vi "Replace Line.vi"(8 "error in":errorcluster, 9 "New Line":T1 {"OPC UA Data Type" items=["Boolean"=1, "SByte"=2, "Byte"=3, "Int16"=4, "UInt16"=5, "Int32"=6, "UInt32"=7, "Int64"=8, "UInt64"=9, "Float"=10, "Double"=11, "String"=12, "DateTime"=13, "ByteString"=15, "Array of Boolean"=101, "Array of SByte"=102, "Array of Byte"=103, "Array of Int16"=104, "Array of UInt16"=105, "Array of Int32"=106, "Array of UInt32"=107, "Array of Int64"=108, "Array of UInt64"=109, "Array of Float"=110, "Array of Double"=111, "Array of String"=112, "Array of DateTime"=113, "Array of ByteString"=115]}, 10 "Line Name":string, 11 "OPC UA configuration in":refnum<class "OPC UA Client configuration.lvclass">) -> (0 "error out":errorcluster, 2 "Old Line":T1 {"OPC UA Data Type" items=["Boolean"=1, "SByte"=2, "Byte"=3, "Int16"=4, "UInt16"=5, "Int32"=6, "UInt32"=7, "Int64"=8, "UInt64"=9, "Float"=10, "Double"=11, "String"=12, "DateTime"=13, "ByteString"=15, "Array of Boolean"=101, "Array of SByte"=102, "Array of Byte"=103, "Array of Int16"=104, "Array of UInt16"=105, "Array of Int32"=106, "Array of UInt32"=107, "Array of Int64"=108, "Array of UInt64"=109, "Array of Float"=110, "Array of Double"=111, "Array of String"=112, "Array of DateTime"=113, "Array of ByteString"=115]}, 3 "OPC UA configuration out":refnum<class "OPC UA Client configuration.lvclass">)   [LabVIEW 2014, in "OPC UA Client configuration.lvclass"]
uses:
  OPC UA Client configuration.lvclass
  Line.ctl
  <vilib>/NI/Tag Bus Module Framework/channel/TBM channel.lvclass
  OPC UA Data Type.ctl
  OPC UA Client configuration.lvclass/OPC UA Client configuration.ctl
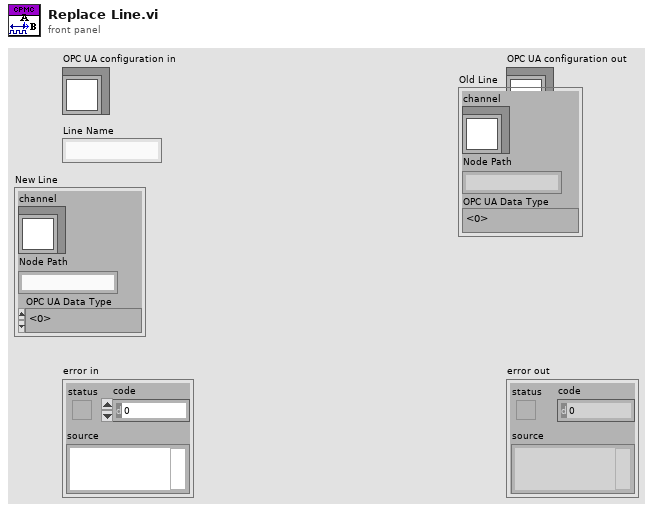
[diagram p1: front panel]
types:
  T1 = typedef "OPC UA Client configuration.lvclass/Line.ctl" = cluster{"channel":refnum<class "TBM channel.lvclass">, "Node Path":string, "OPC UA Data Type":T2}
  T2 = typedef "OPC UA Client configuration.lvclass/OPC UA Data Type.ctl" = u16
  T3 = cluster{"channel":refnum<class "TBM channel.lvclass">, "Node Path":string, "OPC UA Data Type":T2}[]
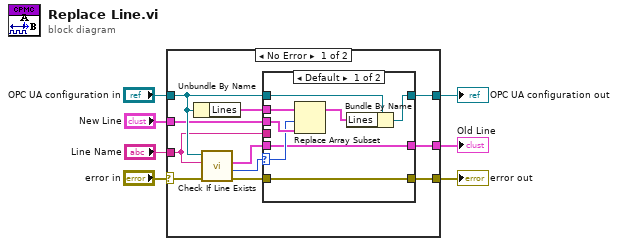
[diagram p0: block diagram]
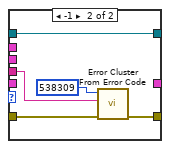
[diagram p2: hidden frame]
diagram:
  n1 = case shown="No Error" "error in" {
    selector: "error in" -> [w10 w33]
    tunnel: [w17 w33] -> w6
    tunnel: [w18 w32] -> w4
    tunnel: "OPC UA configuration in" -> [w16 w32]
    tunnel: "Line Name" -> [w15 _]
    tunnel: "New Line" -> [w13 _]
    tunnel: [w11 _] -> w1
    frame No Error {
      n2 = Unbundle By Name(w16) -> ("Lines"=w12:T3)
      n3 = call-dynamic "Check If Line Exists.vi"("error in"=w10, "name to locate"=w15, "OPC UA configuration in"=w16) -> ("error out"=w9:errorcluster, "index"=w14:i32, "Line out"=w8:T1)  [unwired: 4 in, 2 out]
      n4 = case shown="Default" w14 {
        selector: w14 -> [w20 _]
        tunnel: w16 -> [w26 w31]
        tunnel: [w25 w31] -> w18
        tunnel: w12 -> [w21 _]
        tunnel: w13 -> [w23 _]
        tunnel: w15 -> [_ w29]
        tunnel: w9 -> [w22 w28]
        tunnel: [w22 w27] -> w17
        tunnel: [w19 _] -> w11
        tunnel: w8 -> [w19 _]
        frame Default {
          n5 = Replace Array Subset(array=w21, new element=w23, index=w20) -> (w24:T3)
          n6 = Bundle By Name(cluster=w26, "Lines"=w24) -> (w25:refnum<class "OPC UA Client configuration.lvclass">)
        }
        frame -1 {
          n7 = call <vilib>:"Error Cluster From Error Code.vi"("error in (no error)"=w28, "error message (\"\")"=w29, "error code (0)"=538309) -> ("error out"=w27:errorcluster)  [unwired: 6 in]
        }
      }
    }
    frame Error {
    }
  }
  "error out" <- w6
  "OPC UA configuration out" <- w4
  "Old Line" <- w1
